vi "ToString.vi"(8 "error in (no error)":errorcluster, 11 "StringContains in":refnum<class "StringContains.lvclass">) -> (0 "error out":errorcluster, 2 "String":string, 3 "StringContains out":refnum<class "StringContains.lvclass">)   [LabVIEW 2019, in "Constraint.lvlib" / "StringContains.lvclass"]
doc: "Returns a string representation of the object."
uses:
  StringContains.lvclass
  StringContains.lvclass/StringContains.ctl
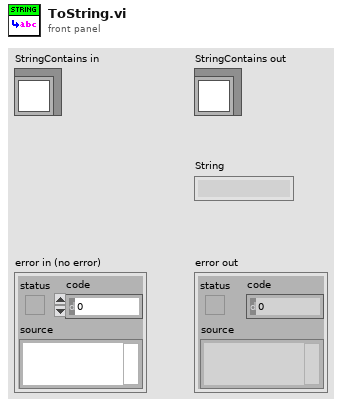
[diagram p1: front panel]
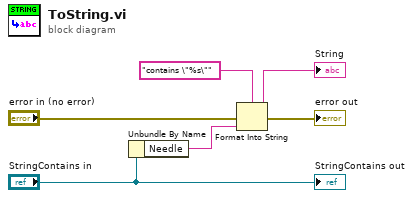
[diagram p0: block diagram]
diagram:
  n1 = Unbundle By Name("StringContains in") -> ("Needle"=w2:string)
  n2 = Format Into String(format string="contains \"%s\"", error in="error in (no error)", w2) -> (resulting string=→"String":string, error out=→"error out":errorcluster)  [unwired: 1 in]
  "StringContains out" <- "StringContains in"
